vi "Scan for timestamp.vi"(9 "Row Index":i32, 10 "Item Names":string[][](array[string]), 11 "Column Headers":string[](array[string])) -> (1 "found":bool, 2 "Time Stamp":timestamp)   [LabVIEW 2019, in "Report Viewer.lvlib" / "Report Viewer.lvclass"]
uses:
  Library/Report Viewer.lvclass
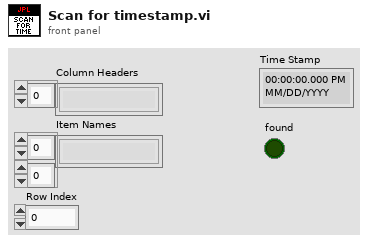
[diagram p1: front panel]
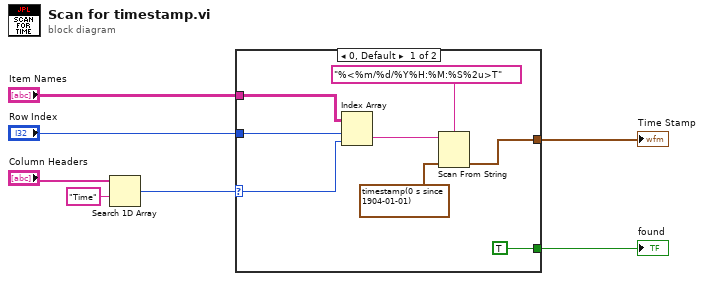
[diagram p0: block diagram]
diagram:
  n1 = Search 1D Array(1D array="Column Headers", element="Time") -> (index of element=w5:i32)  [unwired: 1 in]
  n2 = case shown="0, Default" w5 {
    selector: w5 -> [w14 _]
    tunnel: "Item Names" -> [w15 _]
    tunnel: "Row Index" -> [w13 _]
    tunnel: [w10 _] -> w2
    tunnel: [TRUE _] -> w1
    frame 0, Default {
      n3 = Index Array(array=w15, index (row)=w13, index (col)=w14) -> (element=w12:string)
      n4 = Scan From String(format string="%<%m/%d/%Y%H:%M:%S%2u>T", input string=w12, default 1=timestamp(0 s since 1904-01-01) ("Time Stamp")) -> (output 1=w10:timestamp)  [unwired: 2 in, 3 out]
    }
    frame -1 {
    }
  }
  "found" <- w1
  "Time Stamp" <- w2
